vi "zadanie4_subvi.vi"(8 "error in (no error)":errorcluster, 9 "continue":bool, 10 "Wpisz hasło:":string, 11 "Wpisz login:":string) -> (0 "error out":errorcluster, 2 "hasło:out":string, 3 "login:out":string)   [LabVIEW 2020]
panel:
  # "zaloguj się aby rozpocząć"
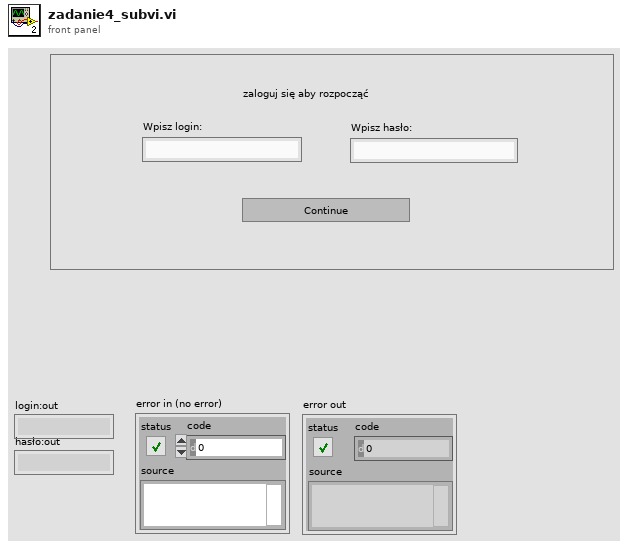
[diagram p1: front panel]
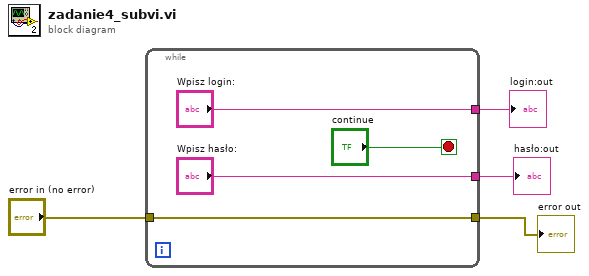
[diagram p0: block diagram]
diagram:
  n1 = while {
    tunnel: ["Wpisz login:"] -> w3
    tunnel: ["Wpisz hasło:"] -> w4
    tunnel: [w5] -> w2
    tunnel: "error in (no error)" -> [w5]
    stop <- "continue" stop-if-true
  }
  "hasło:out" <- w4
  "login:out" <- w3
  "error out" <- w2
